vi "Receive.vi"(8 "error in (no error)":errorcluster, 10 "Transfer Group in":refnum<class "Transfer Group.lvclass">=refnum, 11 "UDP Transceiver in":refnum<class "UDP Transceiver.lvclass">=refnum) -> (0 "error out":errorcluster, 2 "Transfer Group out":refnum<class "Transfer Group.lvclass">, 3 "UDP Transceiver out":refnum<class "UDP Transceiver.lvclass">)   [LabVIEW 2020, in "UDP.lvlib" / "UDP Transceiver.lvclass"]
uses:
  UDP Transceiver.lvclass
  DSF Core.lvlibp/Classes/Transfer Group/Transfer Group.lvclass
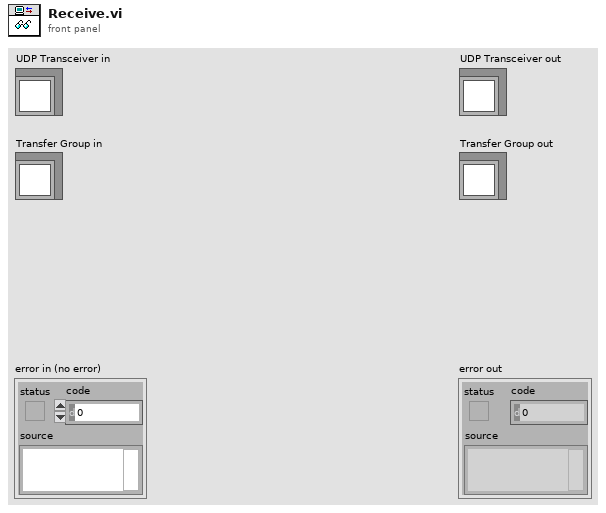
[diagram p1: front panel]
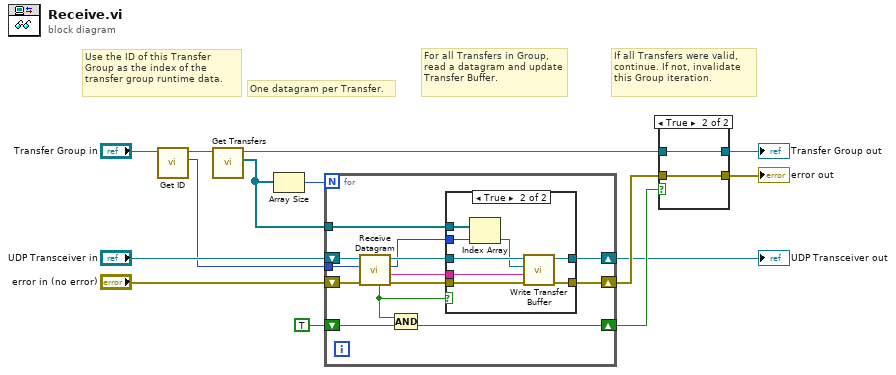
[diagram p0: block diagram]
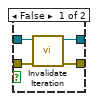
[diagram p3: hidden frame]
diagram:
  # "If all Transfers were valid, continue. If not, invalidate this Group iteration."
  # "Use the ID of this Transfer Group as the index of the transfer group runtime data."
  # "For all Transfers in Group, read a datagram and update Transfer Buffer."
  # "One datagram per Transfer."
  n1 = call "Get ID.vi"("Transfer Group in"="Transfer Group in") -> ("id"=w2:i32, "Transfer Group out"=w14:refnum<class "Transfer Group.lvclass">)  [unwired: 9 in]
  n2 = call "Get Transfers.vi"("Transfer Group in"=w14) -> ("Transfers"=w3:refnum<class "Transfer.lvclass">[], "Transfer Group out"=w5:refnum<class "Transfer Group.lvclass">)  [unwired: 9 in]
  n3 = Array Size(array=w3) -> (size(s)=w13:i32)
  n4 = for {
    N: w13 -> [_]
    shift-right: [w21] -> w11
    shift-left: "error in (no error)" -> [w26]
    shift-right: [w22] -> w1
    shift-left: "UDP Transceiver in" -> [w27]
    tunnel: w2 -> [w18]
    shift-right: [w19] -> w6
    shift-left: TRUE -> [w20]
    tunnel: w3 -> [w15]
    n5 = call "Receive Datagram.vi"("error in (no error)"=w26, "transfer group id"=w18, "UDP Transceiver in"=w27) -> ("error out"=w24:errorcluster, "transfer data"=w23:string, "transfer id"=w17:i32, "UDP Transceiver out"=w25:refnum<class "UDP Transceiver.lvclass">, "valid"=w16:bool)  [unwired: 4 in]
    n6 = Compound Arithmetic op=AND(w16, w20) -> (w19:bool)
    n7 = case shown="True" w16 {
      tunnel: w25 -> [w29 w35]
      tunnel: w24 -> [w28 w34]
      tunnel: w23 -> [_ w33]
      tunnel: [w29 w30] -> w22
      tunnel: [w28 w31] -> w21
      tunnel: w17 -> [_ w36]
      tunnel: w15 -> [_ w37]
      frame False {
      }
      frame True {
        n8 = Index Array(array=w37, index=w36) -> (element=w32:refnum<class "Transfer.lvclass">)
        n9 = call "Write Transfer Buffer.vi"("error in (no error)"=w34, "data"=w33, "Transfer"=w32, "UDP Transceiver in"=w35) -> ("error out"=w31:errorcluster, "UDP Transceiver out"=w30:refnum<class "UDP Transceiver.lvclass">)  [unwired: 6 in]
      }
    }
  }
  "UDP Transceiver out" <- w1
  n10 = case shown="True" w6 {
    tunnel: w11 -> [w41 w43]
    tunnel: [w40 w43] -> w10
    tunnel: w5 -> [w39 w42]
    tunnel: [w38 w42] -> w4
    frame False {
      n11 = call "Invalidate Iteration.vi"("error in (no error)"=w41, "Transfer Group in"=w39) -> ("error out"=w40:errorcluster, "Transfer Group out"=w38:refnum<class "Transfer Group.lvclass">)  [unwired: 8 in]
    }
    frame True {
    }
  }
  "error out" <- w10
  "Transfer Group out" <- w4
